vi "Write Route Manager.vi"(10 "Route Manager.lvclass":refnum<class "slscsl.lvclass">, 11 "SLSC Switch in":refnum<class "SLSC Switch.lvclass">) -> (3 "SLSC Switch out":refnum<class "SLSC Switch.lvclass">)   [LabVIEW 2015, in "SLSC Switch.lvlib" / "SLSC Switch.lvclass"]
uses:
  SLSC Switch.lvclass
  slscsl/slscsl.lvclass
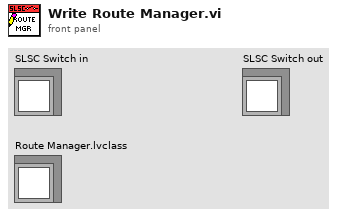
[diagram p1: front panel]
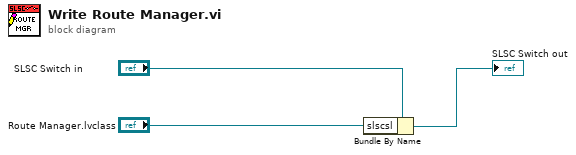
[diagram p0: block diagram]
diagram:
  n1 = Bundle By Name(cluster="SLSC Switch in", "slscsl"="Route Manager.lvclass") -> (→"SLSC Switch out":refnum<class "SLSC Switch.lvclass">)
